vi "Open_Text_Sequence.vi"(0 "Text File":path) -> (1 "Sequence":cluster{string, string[], dbl[], dbl}[](array[cluster]), 2 "Header":string[](array[string]))   [LabVIEW 2011]
doc: "This VI loads and parses a text file containing a growth sequence. Text-based growth sequences are now obsolete, this VI only exists to import old growth sequence files."
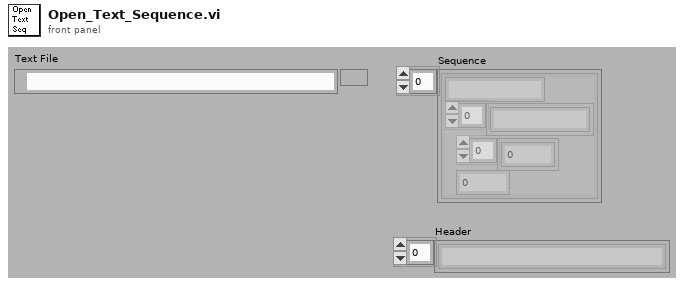
[diagram p1: front panel]
types:
  T1 = cluster{"Command":string, "New Argument List":string[], "Flow Array":dbl[], dbl}[]
  T2 = cluster{"Command":string, "New Argument List":string[], "Flow Array":dbl[], dbl}
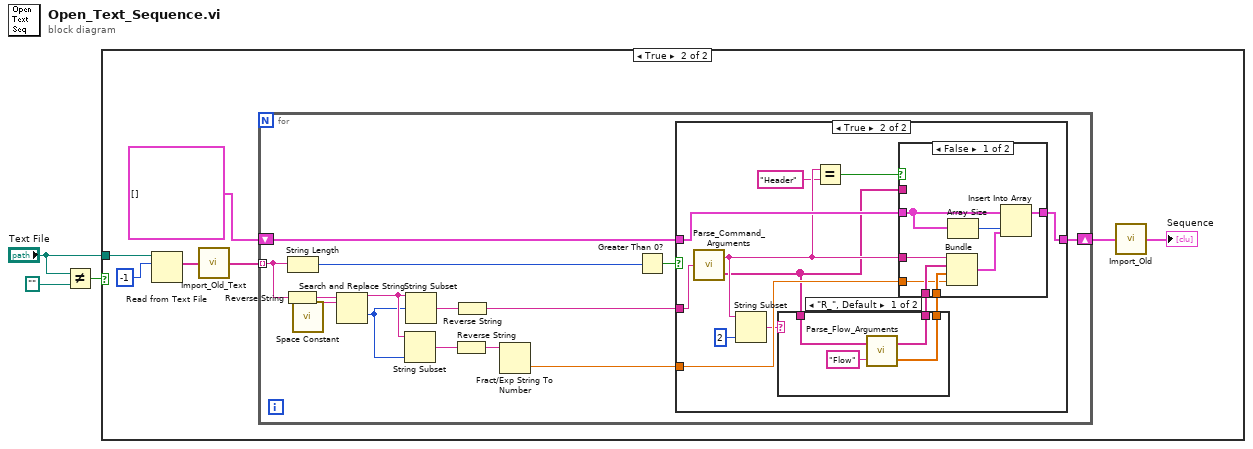
[diagram p0: block diagram]
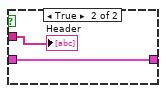
[diagram p4: hidden frame]
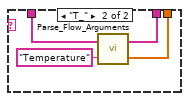
[diagram p5: hidden frame]
diagram:
  n1 = Not Equal?(x="Text File", y=path "") -> (x != y?=w1:bool)
  n2 = case shown="True" w1 {
    tunnel: "Text File" -> [_ w6]
    frame False {
    }
    frame True {
      n3 = Read from Text File(file (use dialog)=w6, count=-1) -> (text=w5:string[])  [unwired: 1 in, 4 out]
      n4 = call "Import_Old_Text.vi"("Input Text"=w5) -> ("Output Text"=w4:string[])
      n5 = for {
        shift-right: [w24] -> w8
        shift-left: T1 [] -> [w23]
        tunnel: w4 -> [w11] mode=indexing
        n6 = Reverse String(1:w11) -> (0:w22:string)
        n7 = String Length(string=w11) -> (length=w12:i32)
        n8 = call <vilib>:"Space Constant.vi"() -> ("String"=w21:string)
        n9 = Search and Replace String(input string=w22, search string=w21) -> (result string=w19:string, offset past replacement=w18:i32)  [unwired: 1 in, 7 out]
        n10 = String Subset(string=w19, length (rest)=w18) -> (substring=w17:string)  [unwired: 1 out]
        n11 = String Subset(string=w19, offset (0)=w18) -> (substring=w20:string)  [unwired: 1 out]
        n12 = Reverse String(1:w17) -> (0:w16:string)
        n13 = Reverse String(1:w20) -> (0:w14:string)
        n14 = Fract/Exp String To Number(string=w16) -> (number=w15:dbl)  [unwired: 4 out]
        n15 = Greater Than 0?(x=w12) -> (x > 0?=w13:bool)
        n16 = case shown="True" w13 {
          tunnel: w14 -> [_ w37]
          tunnel: w15 -> [_ w32]
          tunnel: [w25 w33] -> w24
          tunnel: w23 -> [w25 w34]
          frame False {
          }
          frame True {
            n17 = call "Parse_Command_Arguments.vi"("Command String"=w37) -> ("Command"=w29:string, "Argument List"=w27:string[])
            n18 = String Subset(string=w29, length (rest)=2 ("length (rest)")) -> (substring=w31:string)  [unwired: 1 out]
            n19 = case shown="\"R_\", Default" w31 {
              tunnel: w27 -> [w51 w55]
              tunnel: [w50 w54] -> w36
              tunnel: [w49 w53] -> w35
              frame "R_", Default {
                n20 = call "Parse_Flow_Arguments.vi"("Flow Command String"="Flow", "Argument List"=w51) -> ("Flow Array"=w49:dbl[], "New Argument List"=w50:string[])
              }
              frame "T_" {
                n21 = call "Parse_Flow_Arguments.vi"("Flow Command String"="Temperature", "Argument List"=w55) -> ("Flow Array"=w53:dbl[], "New Argument List"=w54:string[])
              }
            }
            n22 = Equal?(x=w29, y="Header") -> (x = y?=w26:bool)
            n23 = case shown="False" w26 {
              tunnel: w36 -> [w45 _]
              tunnel: w35 -> [w44 _]
              tunnel: w34 -> [w42 w46]
              tunnel: [w40 w46] -> w33
              tunnel: w32 -> [w39 _]
              tunnel: w29 -> [w38 _]
              tunnel: w27 -> [_ w47]
              frame False {
                n24 = Bundle("Command"=w38, "New Argument List"=w45, "Flow Array"=w44, w39) -> (w41:T2)  [unwired: 1 out]
                n25 = Array Size(array=w42) -> (size(s)=w43:i32)
                n26 = Insert Into Array(array=w42, index=w43, new element=w41) -> (w40:T1)
              }
              frame True {
                "Header" <- w47
              }
            }
          }
        }
      }
      n27 = call "Import_Old.vi"("Input Sequence"=w8) -> ("Output Sequence"=→"Sequence":T1)
    }
  }
